vi "DWE Get newest data.vi"(4 "target path":path, 5 "End time":string, 6 "source path":path, 7 "Start time":string, 10 "Previous info":T2={"Last time in range?"=FALSE, "Date"="", "Start index"=1757}, 11 "all rows":string[][](array[string])) -> (2 "New Info":T1, 3 "newest rows":string[][](array[string]))   [LabVIEW 2014]
doc: "Obtain data of one day (instead of entire data sheet for multiple days)."
uses:
  TypeDefs/DWE Data Info.ctl
  <vilib>/Utility/file.llb/Write To Spreadsheet File (string).vi
panel:
  out "concatenated string":string
  out "write path":path
  out "string":string
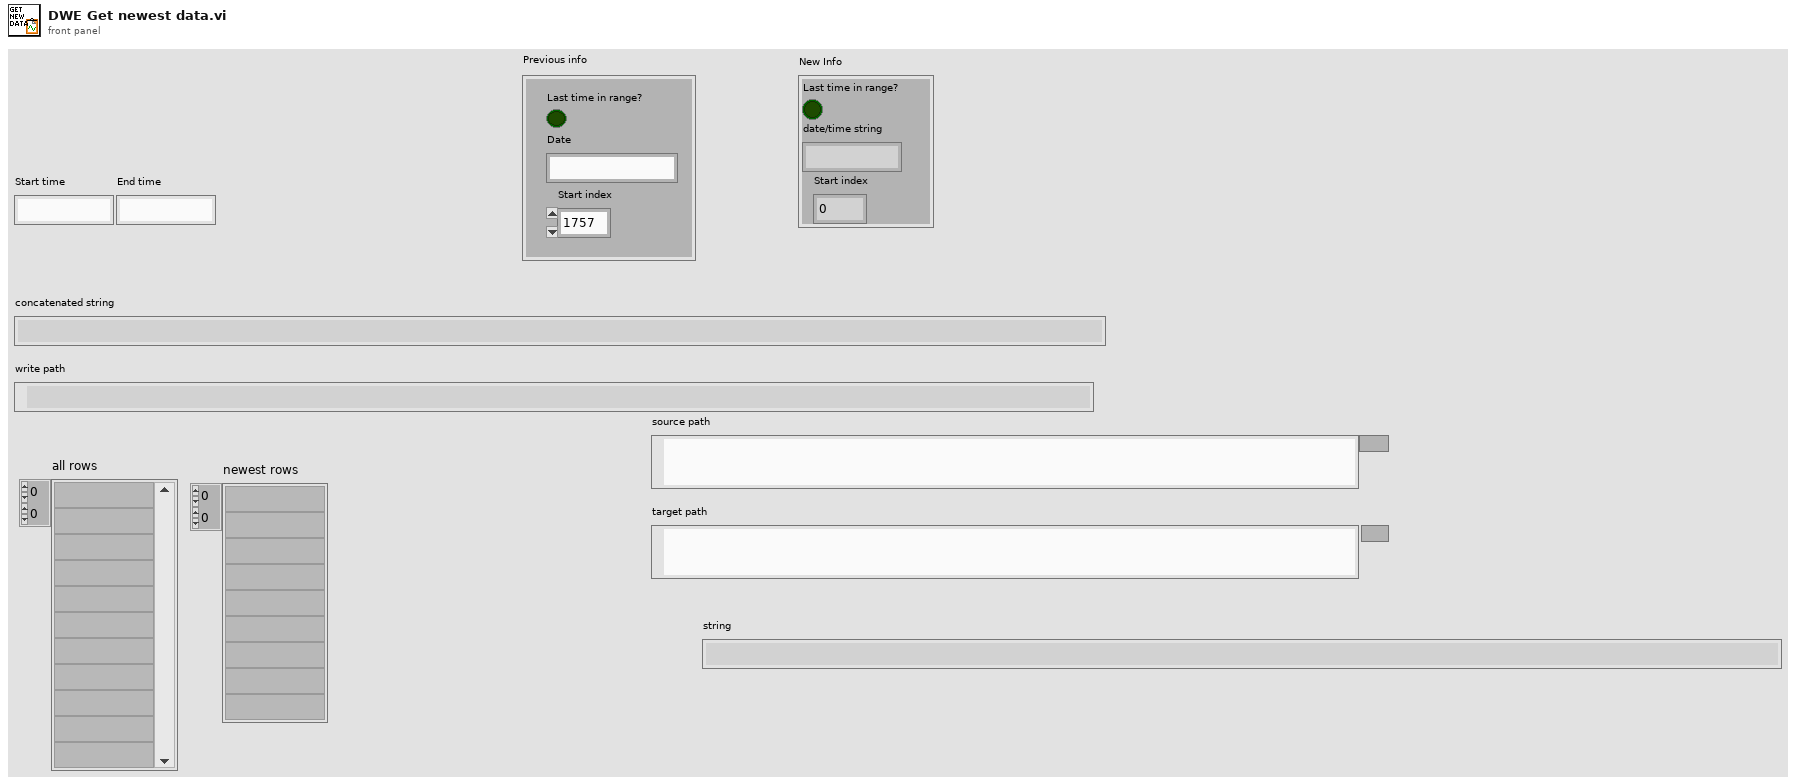
[diagram p1: front panel]
types:
  T1 = cluster{"Last time in range?":bool, "date/time string":string, "Start index":i32}
  T2 = typedef "DWE Data Info.ctl" = cluster{"Last time in range?":bool, "Date":string, "Start index":i32}
  T3 = typedef "LVDateTimeRec.ctl" = cluster{"fractional second":dbl, "second":i32, "minute":i32, "hour":i32, "day of month":i32, "month":i32, "year":i32, "day of week":i32, "day of year":i32, "DST":i32}
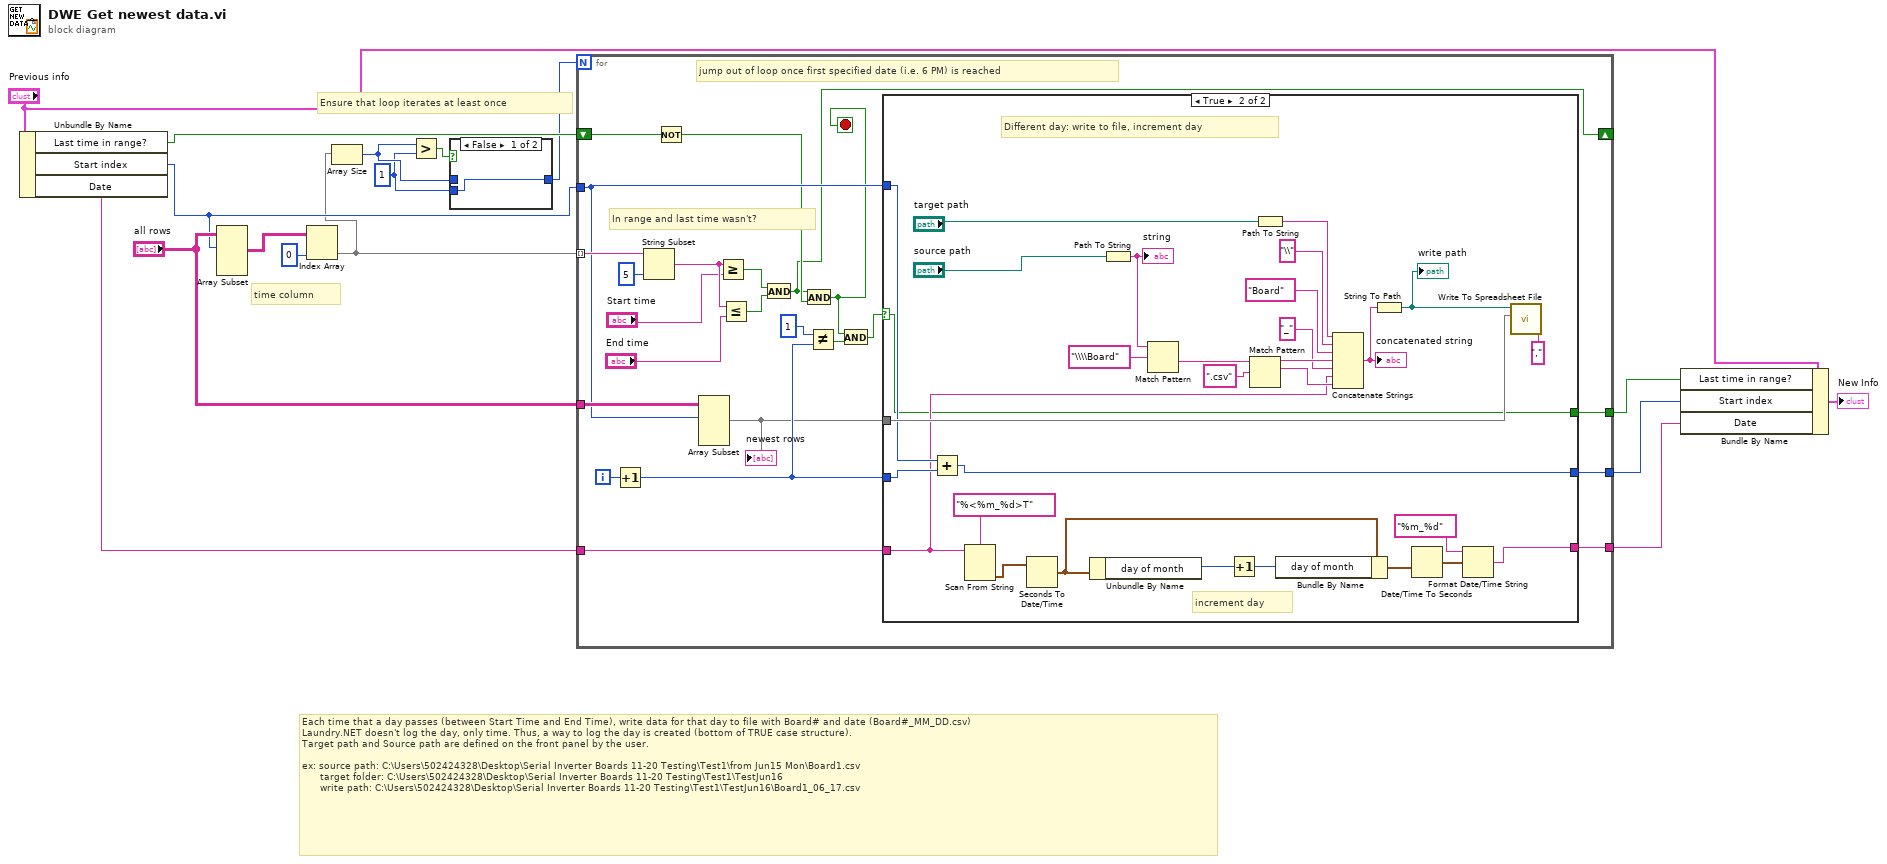
[diagram p0: block diagram]
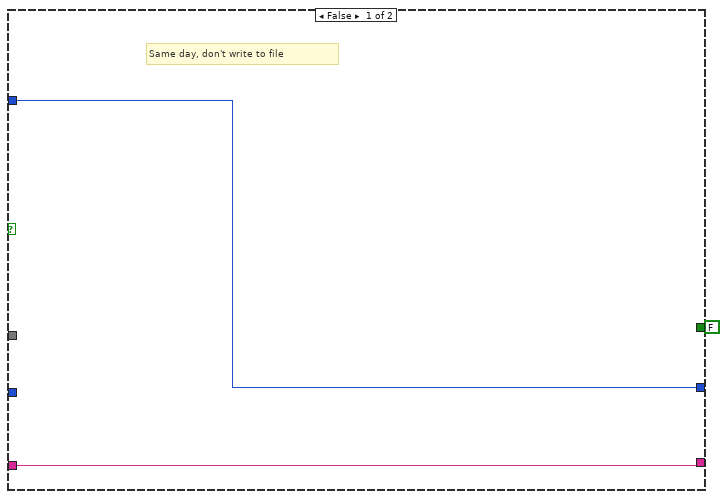
[diagram p3: hidden frame]
diagram:
  w2 = 1 ("y")
  # "Ensure that loop iterates at least once"
  # "time column"
  # "Each time that a day passes (between Start Time and End Time), write data for that day to file with Board# and date (Board#_MM_DD.csv)\nLaundry.NET doesn't log the day, only time. Thus, a way to log the day is created (bottom of TRUE case structure).\nTarget path and Source path are defined on the front panel by the user.\n\nex: source path: C:\\Users\\502424328\\Desktop\\Serial Inverter Boards 11-20 Testing\\Test1\\from Jun15 Mon\\Board1.csv \n      target folder: C:\\Users\\502424328\\Desktop\\Serial Inverter Boards 11-20 Testing\\Test1\\TestJun16\n      write path: C:\\Users\\502424328\\Desktop\\Serial Inverter Boards 11-20 Testing\\Test1\\TestJun16\\Board1_06_17.csv"
  n1 = Unbundle By Name("Previous info") -> ("Last time in range?"=w13:bool, "Start index"=w12:i32, "Date"=w11:string)
  n2 = Array Subset(array="all rows", index (row)=w12) -> (w15:string[][])  [unwired: 3 in]
  n3 = Index Array(array=w15, index (col)=0 ("disabled index (col)")) -> (element=w6:string[])  [unwired: 1 in]
  n4 = Array Size(array=w6) -> (size(s)=w4:i32)
  n5 = Greater?(x=w4, y=w2) -> (0:w5:bool)
  n6 = case shown="False" w5 {
    tunnel: w4 -> [_ w18]
    tunnel: [w17 w18] -> w3
    tunnel: w2 -> [w17 _]
    frame False {
    }
    frame True {
    }
  }
  n7 = for {
    N: w3 -> [_]
    tunnel: w6 -> [w38] mode=indexing
    tunnel: [w37] -> w9
    tunnel: "all rows" -> [w36]
    tunnel: w12 -> [w31]
    tunnel: w11 -> [w30]
    tunnel: [w29] -> w1
    shift-right: [w26] -> _
    shift-left: w13 -> [w28]
    tunnel: [w25] -> w7
    i -> [w35]
    stop <- w24 stop-if-true
    # "In range and last time wasn't?"
    # "jump out of loop once first specified date (i.e. 6 PM) is reached"
    n8 = Increment(x=w35) -> (x+1=w21:i32)
    n9 = String Subset(string=w38, length (rest)=5 ("length (rest)")) -> (substring=w34:string)  [unwired: 1 in]
    n10 = Not(x=w28) -> (.not. x?=w27:bool)
    n11 = Array Subset(array=w36, index (row)=w31) -> (w19:string[][])  [unwired: 3 in]
    "newest rows" <- w19
    n12 = Greater Or Equal?(x=w34, y="Start time") -> (x >= y?=w40:bool)
    n13 = Less Or Equal?(x=w34, y="End time") -> (x <= y?=w39:bool)
    n14 = And(x=w40, y=w39) -> (x .and. y?=w26:bool)
    n15 = And(x=w26, y=w27) -> (x .and. y?=w24:bool)
    n16 = Not Equal?(x=1, y=w21) -> (x != y?=w23:bool)
    n17 = And(x=w24, y=w23) -> (x .and. y?=w22:bool)
    n18 = case shown="True" w22 {
      selector: w22 -> [_ w45]
      tunnel: [w44 w57] -> w37
      tunnel: w19 -> [_ w60]
      tunnel: w31 -> [w44 w59]
      tunnel: w21 -> [_ w58]
      tunnel: w30 -> [w43 w47]
      tunnel: [w43 w48] -> w29
      tunnel: [FALSE w45] -> w25
      frame False {
        # "Same day, don't write to file"
      }
      frame True {
        # "increment day"
        # "Different day: write to file, increment day"
        n19 = Add(x=w59, y=w58) -> (x+y=w57:i32)
        n20 = Scan From String(format string="%<%m_%d>T", input string=w47) -> (output 1=w55:timestamp)  [unwired: 3 in, 3 out]
        n21 = Seconds To Date/Time(time stamp (now)=w55) -> (date time rec=w53:T3)  [unwired: 1 in]
        n22 = Unbundle By Name(w53) -> ("day of month"=w54:i32)
        n23 = Path To String(path="source path") -> (string=w63:string)
        "string" <- w63
        n24 = Match Pattern(string=w63, regular expression="\\\\Board") -> (after substring=w71:string)  [unwired: 1 in, 3 out]
        n25 = Increment(x=w54) -> (x+1=w52:i32)
        n26 = Match Pattern(string=w71, regular expression=".csv") -> (before substring=w69:string, match substring=w67:string)  [unwired: 1 in, 2 out]
        n27 = Path To String(path="target path") -> (string=w72:string)
        n28 = Bundle By Name(cluster=w53, "day of month"=w52) -> (w51:T3)
        n29 = Concatenate Strings(w72, "\\" ("string"), "Board" ("string"), w69, "_" ("string"), w47, w67) -> (w73:string)
        "concatenated string" <- w73
        n30 = String To Path(string=w73) -> (path=w74:path)
        "write path" <- w74
        n31 = Date/Time To Seconds(2:w51) -> (0:w50:timestamp)  [unwired: 1 in]
        n32 = Format Date/Time String(time format string (%c)="%m_%d", seconds (now)=w50) -> (date/time string=w48:string)  [unwired: 1 in]
        n33 = call-poly <vilib>:"Write To Spreadsheet File.vi"("delimiter (\\t)"="," ("delimiter (\\t)"), "2D data"=w60, "file path (dialog if empty)"=w74) -> ()  [unwired: 5 in, 1 out]
      }
    }
  }
  n34 = Bundle By Name(cluster="Previous info", "Last time in range?"=w7, "Start index"=w9, "Date"=w1) -> (→"New Info":T2)
